vi "Amp Filter (SubVI).vi"(6 "Min Frequency":dbl, 9 "Min Amplitude":dbl, 10 "magnitude":dbl[](array[numeric]), 11 "df":dbl) -> (3 "Array":cluster{dbl, "Numeric":dbl}[](array[cluster]))   [LabVIEW 2017]
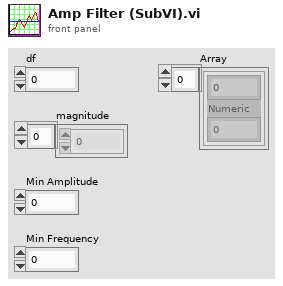
[diagram p1: front panel]
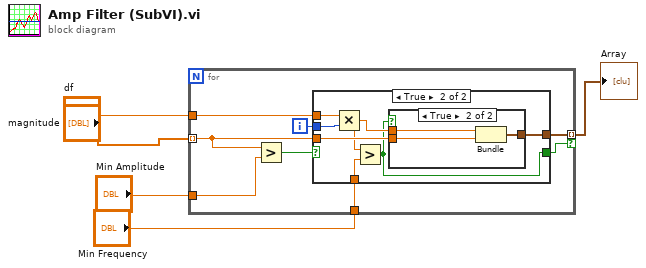
[diagram p0: block diagram]
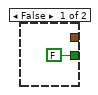
[diagram p2: hidden frame]
diagram:
  n1 = for {
    tunnel: "magnitude" -> [w11] mode=indexing
    tunnel: "df" -> [w13]
    tunnel: [w10] -> w5 mode=indexing if=w6
    tunnel: "Min Amplitude" -> [w9]
    tunnel: "Min Frequency" -> [w8]
    i -> [w12]
    n2 = Greater?(x=w11, y=w9) -> (0:w7:bool)
    n3 = case shown="True" w7 {
      tunnel: w13 -> [_ w21]
      tunnel: w12 -> [_ w18]
      tunnel: w11 -> [_ w19]
      tunnel: [_ w20] -> w10
      tunnel: w8 -> [_ w16]
      tunnel: [FALSE w15] -> w6
      frame False {
      }
      frame True {
        n4 = Multiply(x=w21, y=w18) -> (x*y=w17:dbl)
        n5 = Greater?(x=w17, y=w16) -> (0:w15:bool)
        n6 = case shown="True" w15 {
          tunnel: [_ w24] -> w20
          tunnel: w17 -> [_ w23]
          tunnel: w19 -> [_ w22]
          frame False {
          }
          frame True {
            n7 = Bundle(w23, "Numeric"=w22) -> (w24:cluster{dbl, "Numeric":dbl})  [unwired: 1 in]
          }
        }
      }
    }
  }
  "Array" <- w5
